vi "t.vi"(8 "error in (no error)":errorcluster, 10 "Data DVR":refnum<data-value>, 11 "Type DVR":refnum<data-value>) -> (0 "error out":errorcluster)   [LabVIEW 2023, in "Message Type.lvclass"]
uses:
  Message Type.lvclass
  Message Data/Message Data.lvclass
panel:
  out "Type DVR Out":refnum<data-value>
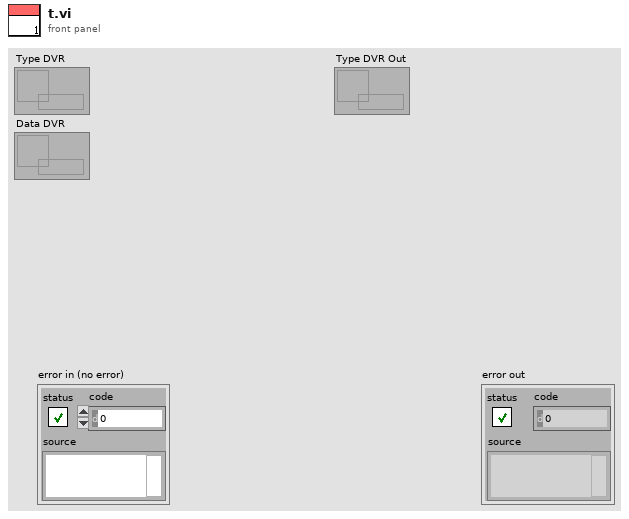
[diagram p1: front panel]
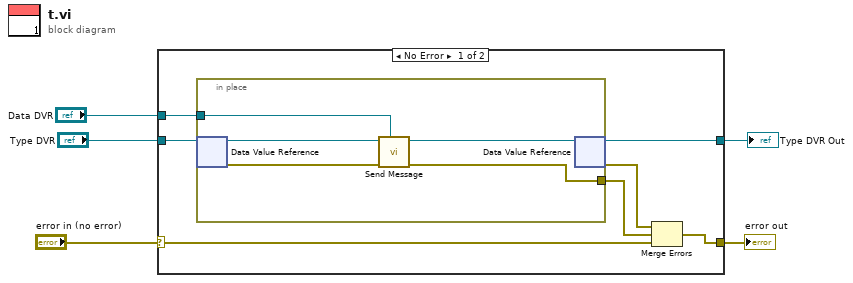
[diagram p0: block diagram]
diagram:
  n1 = case shown="No Error" "error in (no error)" {
    selector: "error in (no error)" -> [w12 w19]
    tunnel: [w8 w19] -> w4
    tunnel: "Type DVR" -> [w11 w18]
    tunnel: "Data DVR" -> [w10 _]
    tunnel: [w9 w18] -> w1
    frame No Error {
      n2 = in-place {
        in-place-border: [w16] -> w7
        in-place-border: w10 -> [w13]
        n3 = in-place-dvr #1(w11) -> (w15:refnum<class "Message Type.lvclass">, w17:errorcluster)
        n4 = call-dynamic "Send Message.vi"("Data DVR"=w13, "error in (no error)"=w17, "Message Type in"=w15) -> ("error out"=w16:errorcluster, "Message Type out"=w14:refnum<class "Message Type.lvclass">)  [unwired: 7 in]
        n5 = in-place-dvr #1(w14) -> (w9:refnum<data-value>, w6:errorcluster)
      }
      n6 = Merge Errors(w6, w7, w12) -> (w8:errorcluster)
    }
    frame Error {
    }
  }
  "error out" <- w4
  "Type DVR Out" <- w1
